vi "Trapeziodal Velocity Control (1).vi"(0 "Active Speed Control Case":T1(ring), 1 "Vmax (mm/s)":dbl, 2 "Accel Rate (mm/s^2)":dbl, 3 "Decel Rate (mm/s^2) 2":dbl, 5 "Current Speed (mm/s)":dbl, 7 "Target Distance (mm)":dbl, 9 "Actual Distance (mm)":dbl, 10 "Creep  Distance (mm)":dbl, 12 "Vcreep (mm/s)":dbl, 13 "Overrun Distance (mm)":dbl, 14 "Timestep (dt)":dbl, 15 "stop or error":bool) -> (4 "Selected Speed Control Case":T1(ring), 6 "Speed Command (mm/s)":dbl)   [LabVIEW 2013]
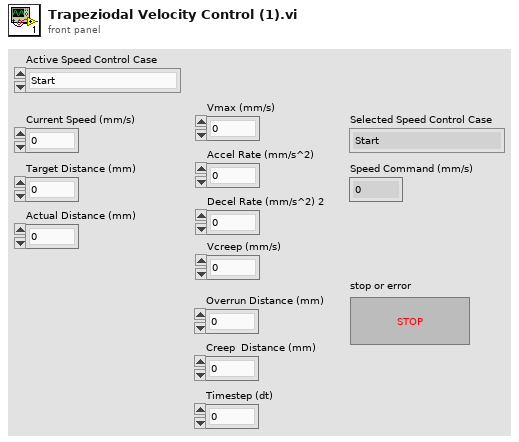
[diagram p1: front panel]
types:
  T1 = enum16{"Start", "Accelerate", "Hold Vmax", "Decelerate", "Hold at Vcreep", "Stop"}
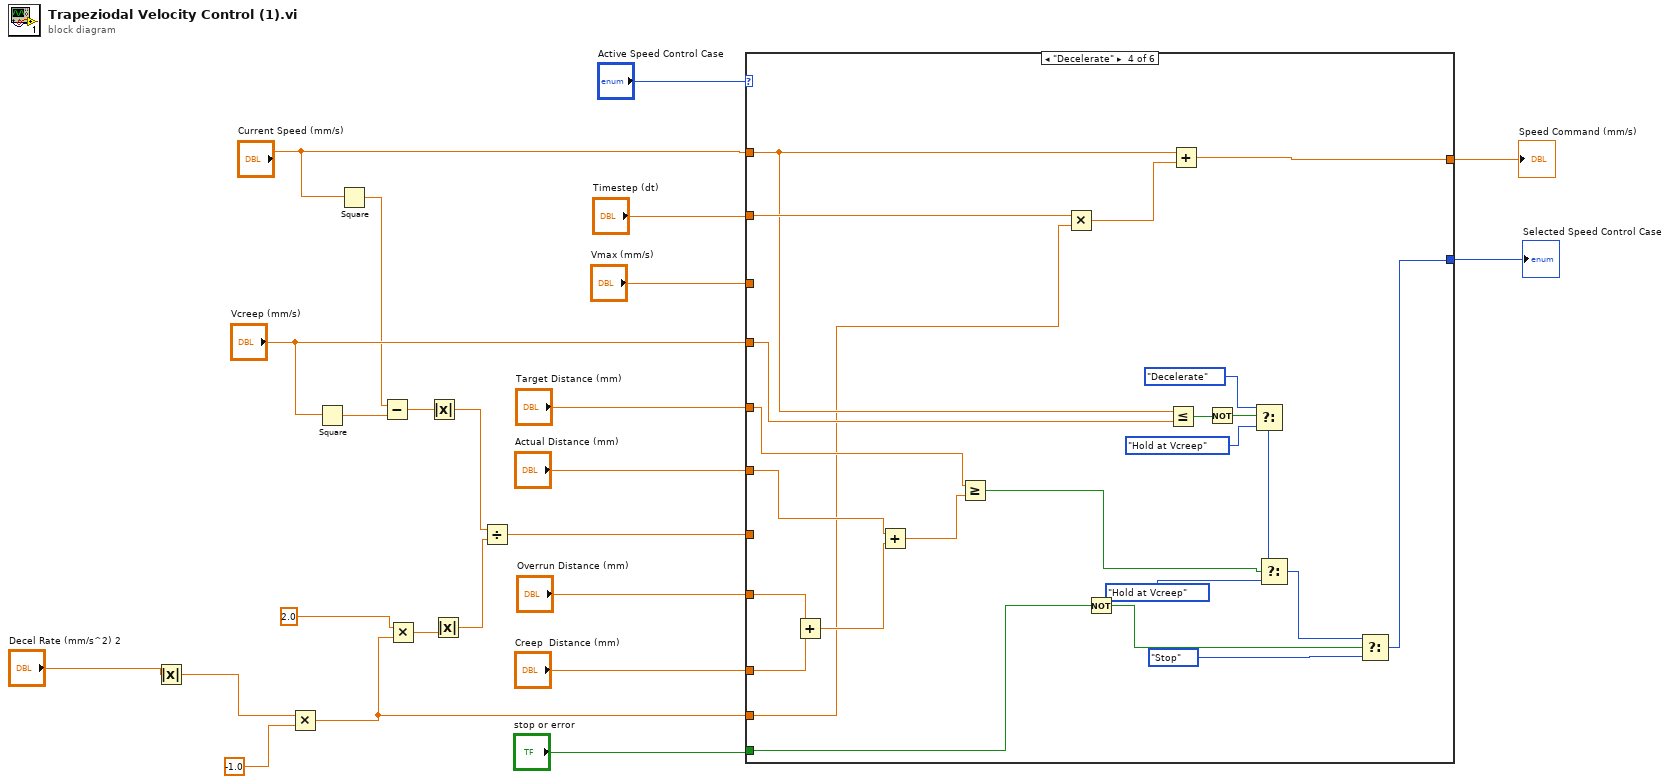
[diagram p0: block diagram]
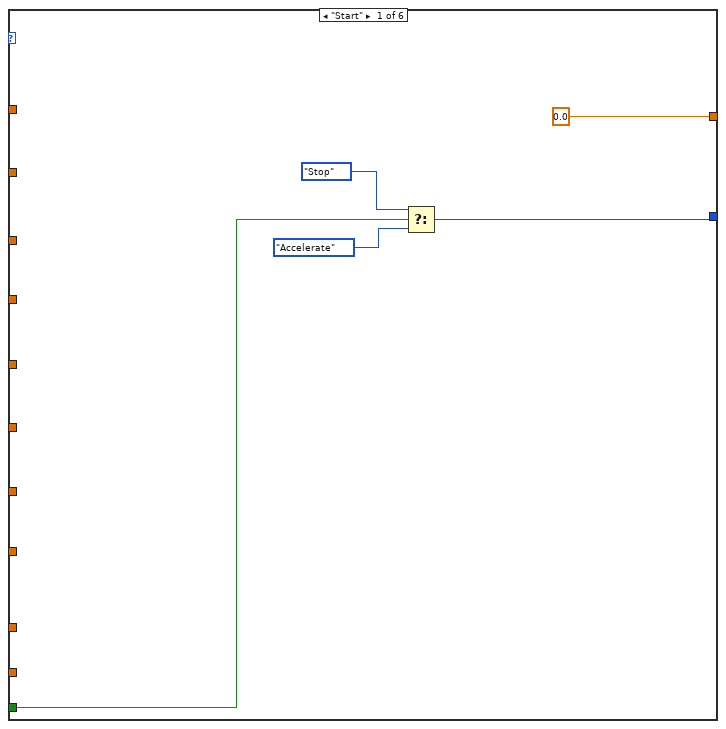
[diagram p2: hidden frame]
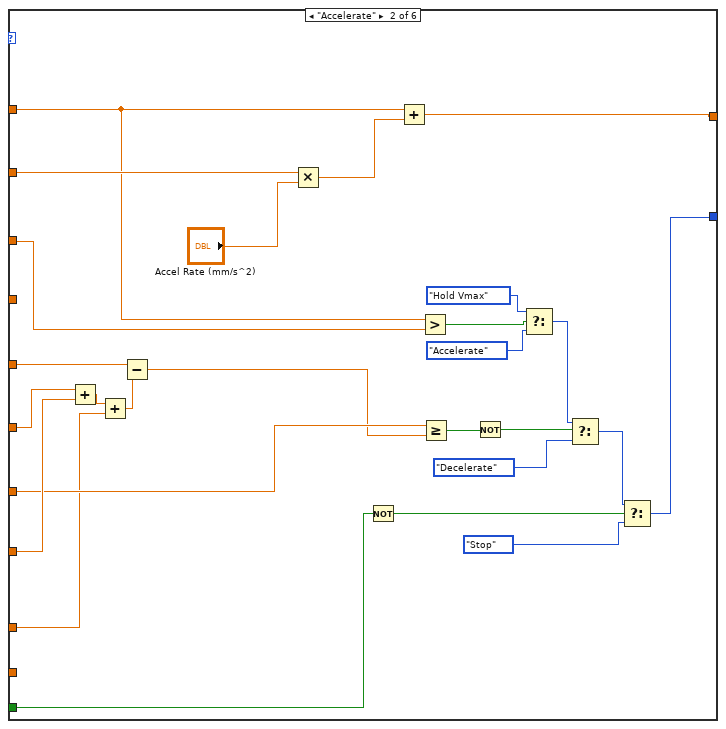
[diagram p3: hidden frame]
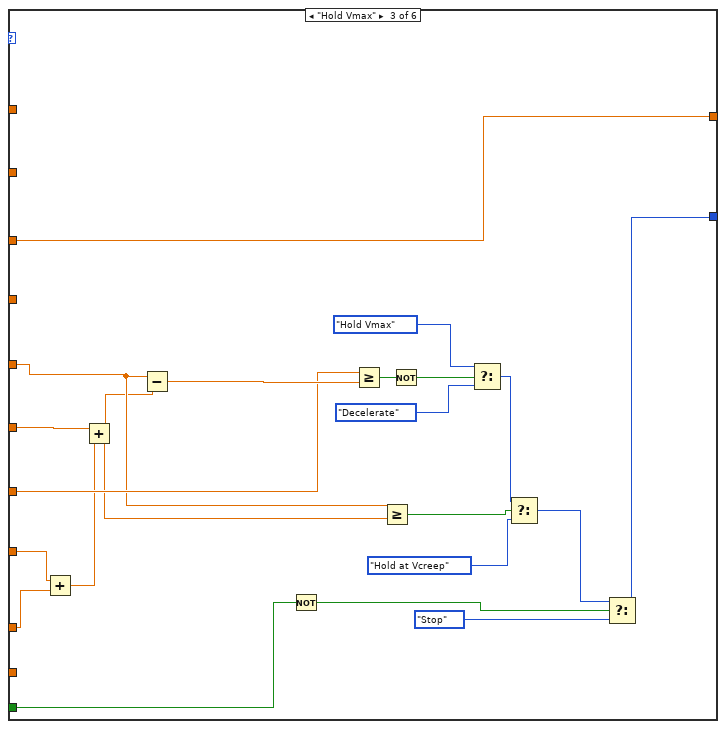
[diagram p4: hidden frame]
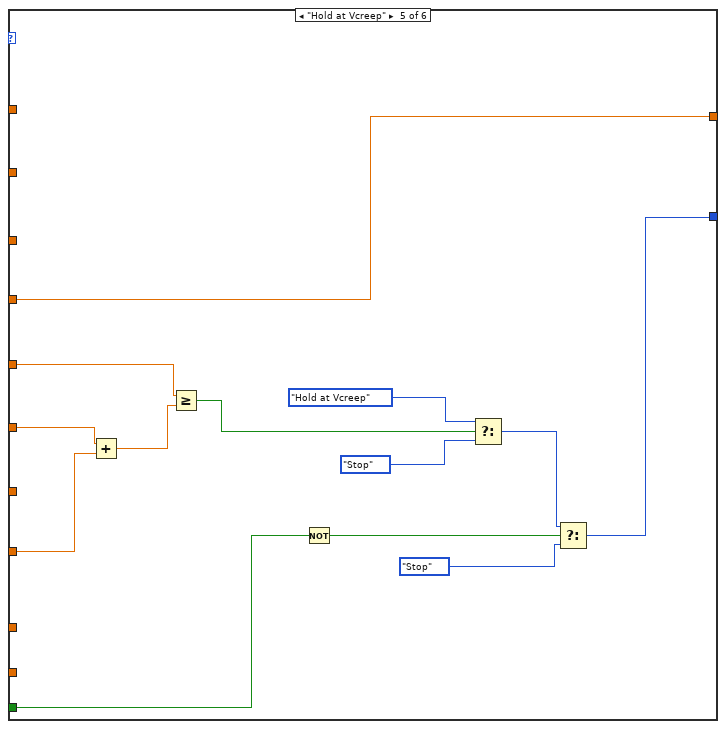
[diagram p5: hidden frame]
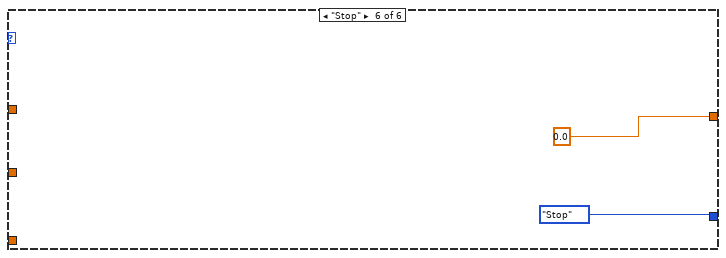
[diagram p6: hidden frame]
diagram:
  n1 = Absolute Value(x="Decel Rate (mm/s^2) 2") -> (abs(x)=w11:dbl)
  n2 = Multiply(x=w11, y=-1.0) -> (x*y=w8:dbl)
  n3 = Square(x="Vcreep (mm/s)") -> (x^2=w5:dbl)
  n4 = Square(x="Current Speed (mm/s)") -> (x^2=w6:dbl)
  n5 = Subtract(x=w6, y=w5) -> (x-y=w4:dbl)
  n6 = Multiply(x=2.0, y=w8) -> (x*y=w2:dbl)
  n7 = Absolute Value(x=w4) -> (abs(x)=w3:dbl)
  n8 = Absolute Value(x=w2) -> (abs(x)=w1:dbl)
  n9 = Divide(x=w3, y=w1) -> (x/y=w14:dbl)
  n10 = case shown="\"Decelerate\"" "Active Speed Control Case" {
    tunnel: [0.0 w52 w76 w77 w113 0.0] -> w24
    tunnel: "Current Speed (mm/s)" -> [_ w47 _ w96 _ _]
    tunnel: "Timestep (dt)" -> [_ w53 _ w99 _ _]
    tunnel: "Vmax (mm/s)" -> [_ w48 w76 _ _ _]
    tunnel: "Vcreep (mm/s)" -> [_ _ _ w95 w113 _]
    tunnel: "stop or error" -> [w28 w42 w73 w87 w110 _]
    tunnel: "Target Distance (mm)" -> [_ w39 w64 w89 w103 _]
    tunnel: w14 -> [_ w36 w67 _ _ _]
    tunnel: "Actual Distance (mm)" -> [_ w38 w68 w88 w105 _]
    tunnel: [w25 w40 w70 w97 w109 T1."Stop" ("Enum 2")] -> w17
    tunnel: "Overrun Distance (mm)" -> [_ w37 w58 w81 w104 _]
    tunnel: "Creep  Distance (mm)" -> [_ w30 w57 w80 _ _]
    tunnel: w8 -> [_ _ _ w78 _ _]
    frame "Start" {
      n11 = Select(t=T1."Stop" ("Enum 2"), s=w28, f=T1."Accelerate" ("Enum 2")) -> (s? t:f=w25:T1)
    }
    frame "Accelerate" {
      n12 = Add(x=w38, y=w37) -> (x+y=w32:dbl)
      n13 = Add(x=w32, y=w30) -> (x+y=w31:dbl)
      n14 = Subtract(x=w39, y=w31) -> (x-y=w35:dbl)
      n15 = Multiply(x=w53, y="Accel Rate (mm/s^2)") -> (x*y=w55:dbl)
      n16 = Not(x=w42) -> (.not. x?=w44:bool)
      n17 = Add(x=w47, y=w55) -> (x+y=w52:dbl)
      n18 = Greater?(x=w47, y=w48) -> (0:w50:bool)
      n19 = Greater Or Equal?(x=w36, y=w35) -> (x >= y?=w34:bool)
      n20 = Not(x=w34) -> (.not. x?=w33:bool)
      n21 = Select(t=T1."Hold Vmax" ("Enum 2"), s=w50, f=T1."Accelerate" ("Enum 2")) -> (s? t:f=w46:T1)
      n22 = Select(t=w46, s=w33, f=T1."Decelerate" ("Enum 2")) -> (s? t:f=w43:T1)
      n23 = Select(t=w43, s=w44, f=T1."Stop" ("Enum 2")) -> (s? t:f=w40:T1)
    }
    frame "Hold Vmax" {
      n24 = Add(x=w58, y=w57) -> (x+y=w56:dbl)
      n25 = Add(x=w68, y=w56) -> (x+y=w63:dbl)
      n26 = Subtract(x=w64, y=w63) -> (x-y=w69:dbl)
      n27 = Not(x=w73) -> (.not. x?=w75:bool)
      n28 = Greater Or Equal?(x=w67, y=w69) -> (x >= y?=w66:bool)
      n29 = Greater Or Equal?(x=w64, y=w63) -> (x >= y?=w60:bool)
      n30 = Not(x=w66) -> (.not. x?=w65:bool)
      n31 = Select(t=T1."Hold Vmax" ("Enum 2"), s=w65, f=T1."Decelerate" ("Enum 2")) -> (s? t:f=w62:T1)
      n32 = Select(t=w62, s=w60, f=T1."Hold at Vcreep" ("Enum 2")) -> (s? t:f=w61:T1)
      n33 = Select(t=w61, s=w75, f=T1."Stop" ("Enum 2")) -> (s? t:f=w70:T1)
    }
    frame "Decelerate" {
      n34 = Add(x=w81, y=w80) -> (x+y=w79:dbl)
      n35 = Add(x=w88, y=w79) -> (x+y=w90:dbl)
      n36 = Greater Or Equal?(x=w89, y=w90) -> (x >= y?=w83:bool)
      n37 = Multiply(x=w99, y=w78) -> (x*y=w100:dbl)
      n38 = Not(x=w87) -> (.not. x?=w86:bool)
      n39 = Less Or Equal?(x=w96, y=w95) -> (x <= y?=w94:bool)
      n40 = Add(x=w96, y=w100) -> (x+y=w77:dbl)
      n41 = Not(x=w94) -> (.not. x?=w93:bool)
      n42 = Select(t=T1."Decelerate" ("Enum 2"), s=w93, f=T1."Hold at Vcreep" ("Enum 2")) -> (s? t:f=w84:T1)
      n43 = Select(t=w84, s=w83, f=T1."Hold at Vcreep" ("Enum 2")) -> (s? t:f=w85:T1)
      n44 = Select(t=w85, s=w86, f=T1."Stop" ("Enum 2")) -> (s? t:f=w97:T1)
    }
    frame "Hold at Vcreep" {
      n45 = Add(x=w105, y=w104) -> (x+y=w102:dbl)
      n46 = Greater Or Equal?(x=w103, y=w102) -> (x >= y?=w101:bool)
      n47 = Not(x=w110) -> (.not. x?=w112:bool)
      n48 = Select(t=T1."Hold at Vcreep" ("Enum 2"), s=w101, f=T1."Stop" ("Enum 2")) -> (s? t:f=w106:T1)
      n49 = Select(t=w106, s=w112, f=T1."Stop" ("Enum 2")) -> (s? t:f=w109:T1)
    }
    frame "Stop" {
    }
  }
  "Speed Command (mm/s)" <- w24
  "Selected Speed Control Case" <- w17
